vi "Set to JSON.vi"(4 "LVClass Serializer":refnum<class "JSONtext LVClass Serializer.lvclass">, 5 "enable LabVIEW extensions?":bool, 6 "Pretty Print?":bool, 8 "error in (no error)":errorcluster, 11 "Variant":variant) -> (0 "error out":errorcluster, 2 "<JSON>":string)   [LabVIEW 2020, in "JSONtext.lvlib" / "SetMap.lvlib"]
uses:
  <vilib>/JDP Science/JSONtext/support/Set Map/SetMap.lvlib
  <vilib>/JDP Science/JSONtext/LVClass Serializer/JSONtext LVClass Serializer.lvclass
  <vilib>/JDP Science/JDP Science Common Utilities/JDP Utility.lvlib
  <vilib>/JDP Science/JSONtext/JSONtext.lvlib
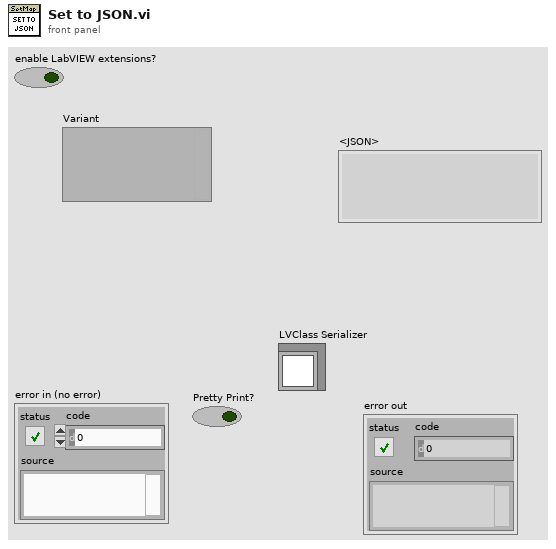
[diagram p1: front panel]
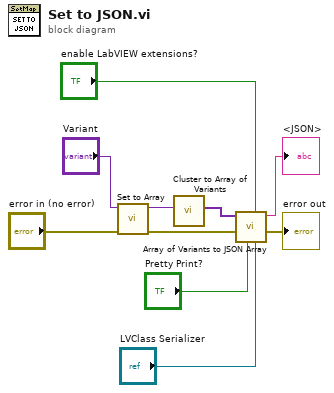
[diagram p0: block diagram]
diagram:
  n1 = call <vilib>:"Set to Array.vi"("error in"="error in (no error)", "Set"="Variant") -> ("error out"=w7:errorcluster, "Array"=w3:variant)  [unwired: 8 in]
  n2 = call <vilib>:"Cluster to Array of Variants.vi"("Cluster"=w3) -> ("Array of Cluster Elements"=w4:variant[])  [unwired: 10 in]
  n3 = call <vilib>:"Array of Variants to JSON Array.vi"("LVClass Serializer"="LVClass Serializer", "enable LabVIEW extensions? (T)"="enable LabVIEW extensions?", "Pretty Print?"="Pretty Print?", "error in (no error)"=w7, "Array of Variants"=w4) -> ("error out"=→"error out":errorcluster, "<JSON>"=→"<JSON>":string)  [unwired: 5 in]
